vi "RunningAverage-GetGroupData.vi"(8 "Error in":errorcluster, 9 "Enabled?":bool, 11 "Device Ref in":T1 format="%.0x") -> (0 "Error out":errorcluster, 2 "Group Data Array":T2(array[cluster]) {"VS Refs" format="%.0x"}, 3 "Device Ref out":T1=18446744073709551615 format="%.0x")   [LabVIEW 2020, in "Waveform-Processing-Custom-Device Shared.lvlib" / "Running Average.lvlib"]
uses:
  Running Average.lvlib
  <vilib>/NI VeriStand/Custom Device API/Custom Device Item Ref.ctl
  Constants.vi
  <vilib>/NI VeriStand/Custom Device API/Get Item Property (Dependent Node Pointer).vi
  <vilib>/NI VeriStand/Custom Device Tools/Custom Device Utility Library/NI VeriStand - Search for Item by GUID.vi
  System Explorer/Waveform-Processing-Custom-Device System Explorer.lvlib
  <vilib>/NI VeriStand/Custom Device API/Custom Device API.lvlib
  Waveform-Processing-Custom-Device Shared.lvlib
  <vilib>/NI VeriStand/Custom Device Tools/Custom Device Utility Library/Custom Device Utility Library.lvlib
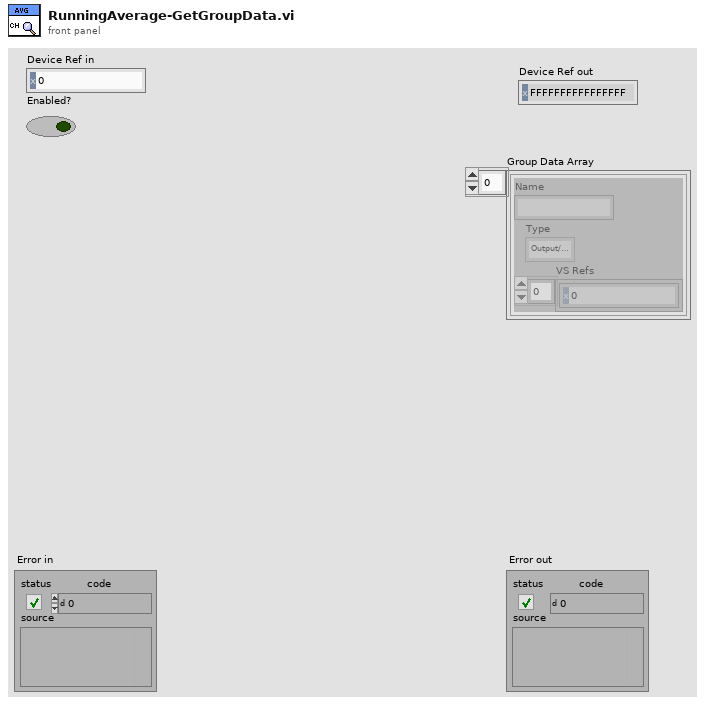
[diagram p1: front panel]
types:
  T1 = typedef "Custom Device API.lvlib/Custom Device Item Ref.ctl" = u64
  T2 = cluster{"Name":string, "Type":enum16{"Output/Write", "Input/Read", "Input/ReadWrite"}, "VS Refs":T1[]}[]
  T3 = enum16{"Output/Write", "Input/Read", "Input/ReadWrite"}
  T4 = cluster{"Name":string, "Type":enum16{"Output/Write", "Input/Read", "Input/ReadWrite"}, "VS Refs":T1[]}
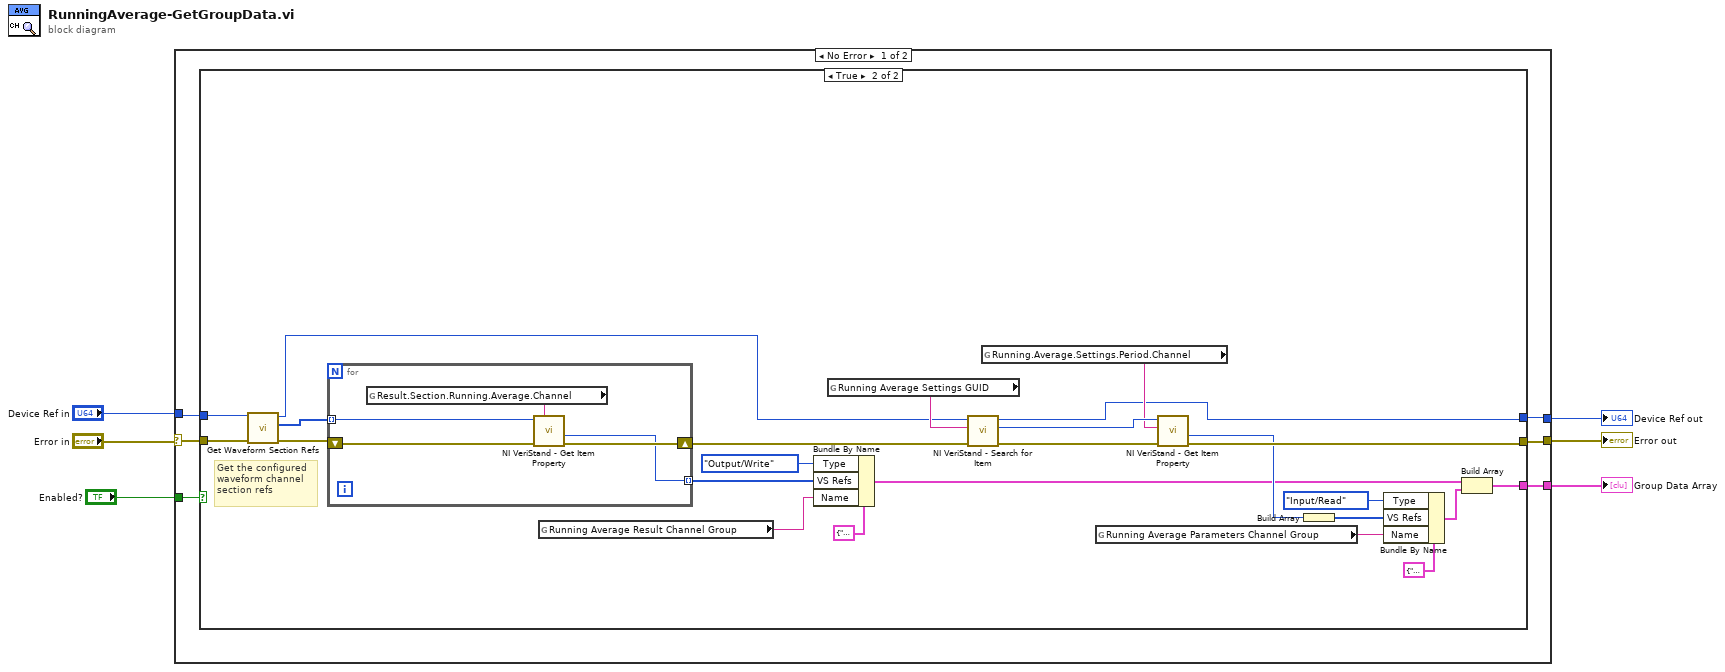
[diagram p0: block diagram]
diagram:
  n1 = case shown="No Error" "Error in" {
    selector: "Error in" -> [w12 w45]
    tunnel: [w10 w45] -> w5
    tunnel: "Device Ref in" -> [w11 w44]
    tunnel: "Enabled?" -> [w9 _]
    tunnel: [w8 w44] -> w2
    tunnel: [w7 _] -> w1
    frame No Error {
      n2 = case shown="True" w9 {
        tunnel: w12 -> [w14 w38]
        tunnel: w11 -> [w13 w36]
        tunnel: [w14 w29] -> w10
        tunnel: [w13 w28] -> w8
        tunnel: [_ w15] -> w7
        frame False {
        }
        frame True {
          # "Get the configured\nwaveform channel\nsection refs"
          n3 = call "Get Waveform Section Refs.vi"("Error in"=w38, "Device Ref in"=w36) -> ("Error out"=w37:errorcluster, "Result Section Refs"=w35:T1[], "Device Ref out"=w26:T1)  [unwired: 7 in]
          n4 = for {
            tunnel: w35 -> [w39] mode=indexing
            shift-right: [w41] -> w34
            shift-left: w37 -> [w43]
            tunnel: [w40] -> w27 mode=indexing
            n5 = global read "Constants.vi" "Result.Section.Running.Average.Channel"() -> (w42:string)
            n6 = call-poly <vilib>:"NI VeriStand - Get Item Property.vi"("error in (no error)"=w43, "Property Name"=w42, "Item Ref in"=w39) -> ("error out"=w41:errorcluster, "Dependent Node Ref"=w40:T1)  [unwired: 5 in, 2 out]
          }
          n7 = global read "Constants.vi" "Running Average Result Channel Group"() -> (w25:string)
          n8 = Bundle By Name(cluster=T4 {"Name"="", "Type"=enum."Output/Write", "VS Refs"=[]} ("Group"), "Type"=T3."Output/Write", "VS Refs"=w27, "Name"=w25) -> (w17:T4)
          n9 = global read "Constants.vi" "Running Average Settings GUID"() -> (w33:string)
          n10 = call-poly <vilib>:"NI VeriStand - Search for Item.vi"("error in"=w34, "Item GUID"=w33, "Section Ref in"=w26) -> ("error out"=w32:errorcluster, "Item Ref"=w31:T1, "Section Ref out"=w28:T1)  [unwired: 5 in, 1 out]
          n11 = global read "Constants.vi" "Running.Average.Settings.Period.Channel"() -> (w30:string)
          n12 = global read "Constants.vi" "Running Average Parameters Channel Group"() -> (w20:string)
          n13 = call-poly <vilib>:"NI VeriStand - Get Item Property.vi"("error in (no error)"=w32, "Property Name"=w30, "Item Ref in"=w31) -> ("error out"=w29:errorcluster, "Dependent Node Ref"=w19:T1)  [unwired: 5 in, 2 out]
          n14 = Build Array(w19) -> (w18:T1[])
          n15 = Bundle By Name(cluster=T4 {"Name"="", "Type"=enum."Output/Write", "VS Refs"=[]} ("Group"), "Type"=T3."Input/Read", "VS Refs"=w18, "Name"=w20) -> (w16:T4)
          n16 = Build Array(w17, w16) -> (w15:T2)
        }
      }
    }
    frame Error {
    }
  }
  "Error out" <- w5
  "Device Ref out" <- w2
  "Group Data Array" <- w1
